vi "General Config.vi"(8 "error In":errorcluster, 10 "IOList":T2, 11 "reference":refnum<vi>) -> (0 "error out":errorcluster, 3 "Out reference":refnum<vi>)   [LabVIEW 2015]
uses:
  Control Button/Exit.ctl
  Control Button/Daq.ctl
  Control Button/Scanner config.ctl
  Control Button/Program Seq.ctl
  Control Button/cali.ctl
  Control Button/shift change.ctl
  Control Button/User mgt.ctl
  Control Button/model create.ctl
  Galobal variable_TI.vi
panel:
  in  "Setting":bool
  in  "image Setting":bool
  out "User Name 3":string
  in  "Model Create":T1
  in  "User Mgt":T3
  out "User Name 2":string
  in  "Shift":T4
  in  "Calibration":T5
  in  "IO List Update":bool
  out "error out 2":errorcluster
  in  "error in (no error)":errorcluster
  in  "Program Seq":T6
  in  "Scanner config":T7
  in  "DAQ Config":T8
  out "User Name":string
  in  "Exit":T9
  out "String":string
  out "appended path":path
  in  "Ring":u16(ring)
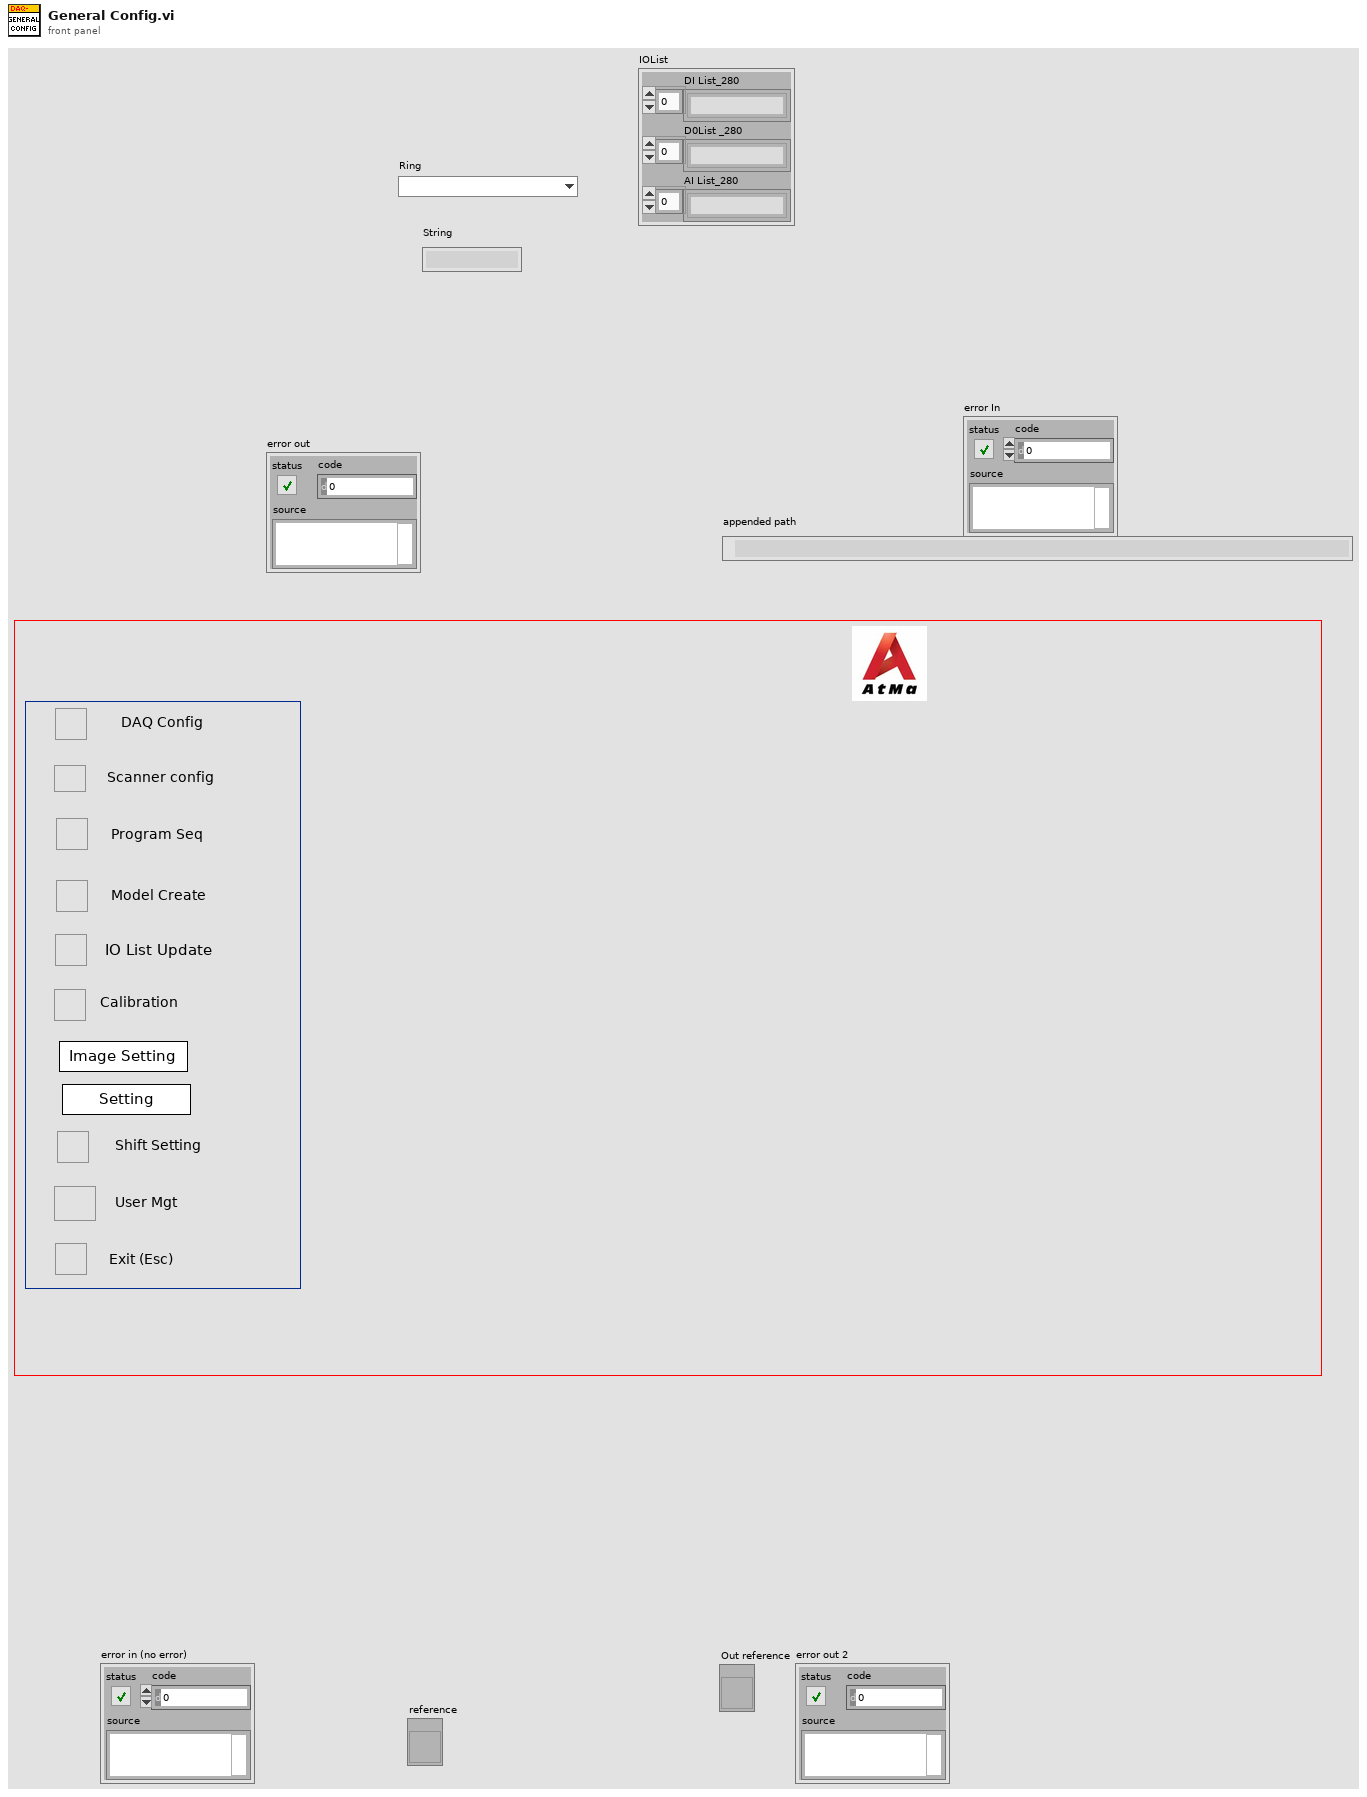
[diagram p1: front panel]
types:
  T1 = typedef "model create.ctl" = bool
  T2 = cluster{"DI List_280":string[], "D0List _280":string[], "AI List_280":string[]}
  T3 = typedef "User mgt.ctl" = bool
  T4 = typedef "shift change.ctl" = bool
  T5 = typedef "cali.ctl" = bool
  T6 = typedef "Program Seq.ctl" = bool
  T7 = typedef "Scanner config.ctl" = bool
  T8 = typedef "Daq.ctl" = bool
  T9 = typedef "Exit.ctl" = bool
  T10 = enum32{"Invalid", "Standard", "Closed", "Hidden", "Minimized", "Maximized"}
  T11 = cluster{"XInput":dbl[], "Y New Value":dbl[], "Avg point":i16}[]
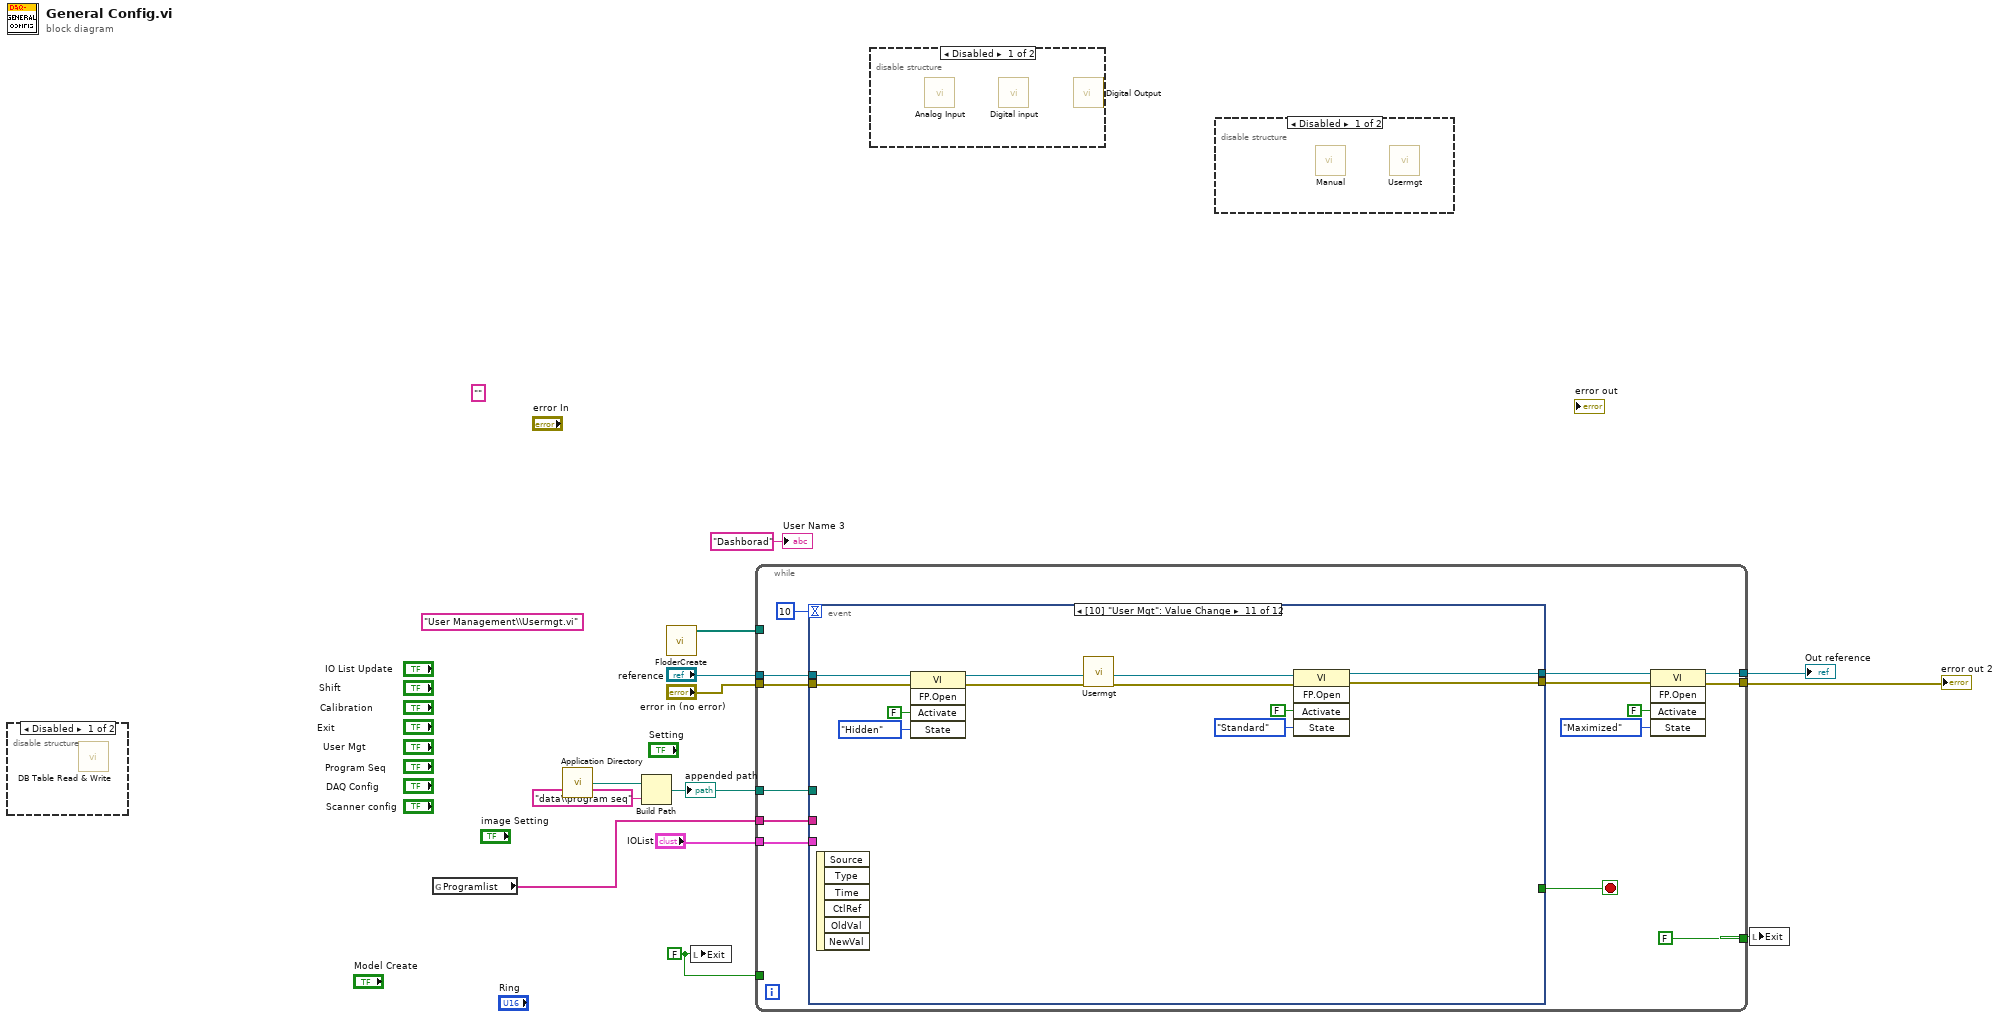
[diagram p0: block diagram]
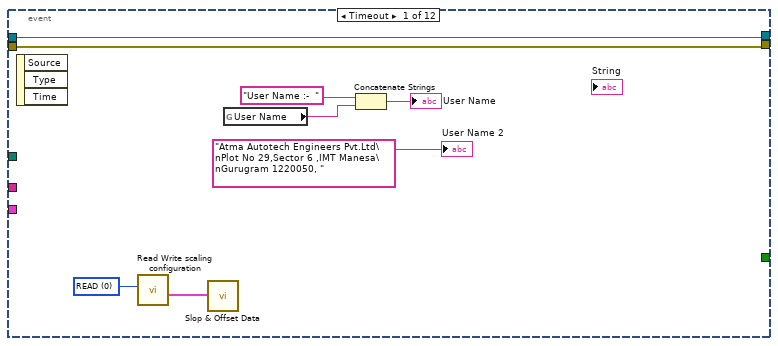
[diagram p5: hidden frame]
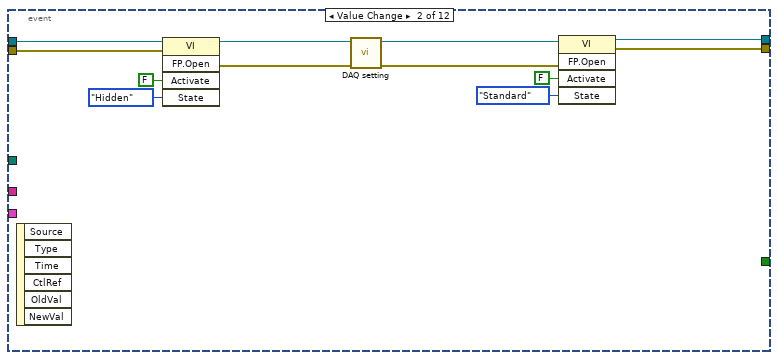
[diagram p6: hidden frame]
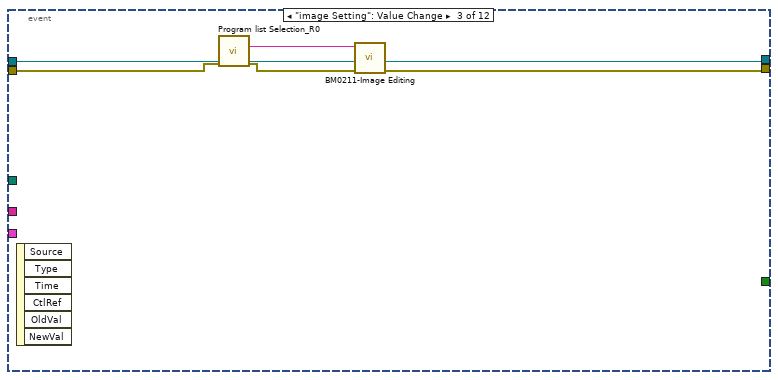
[diagram p7: hidden frame]
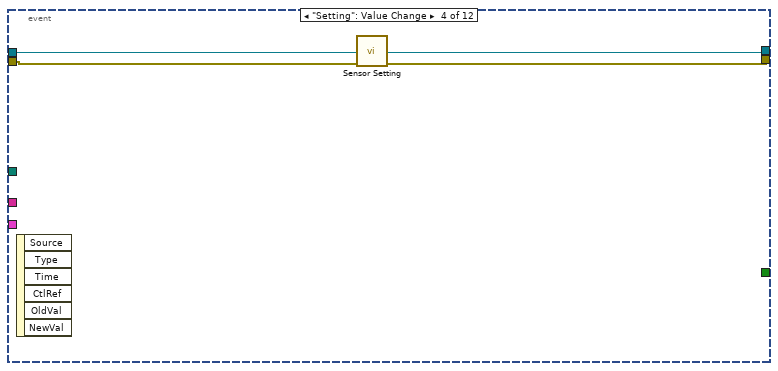
[diagram p8: hidden frame]
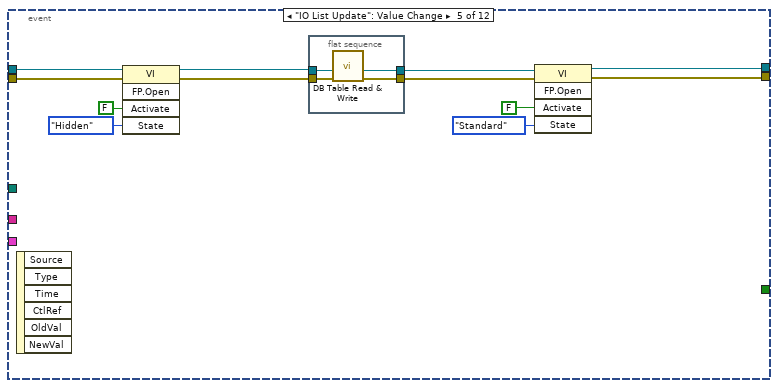
[diagram p9: hidden frame]
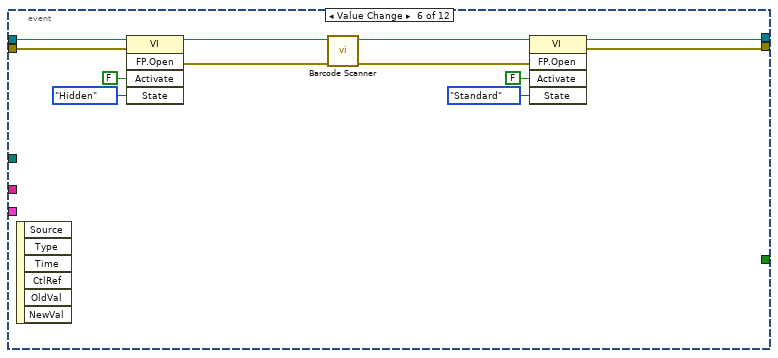
[diagram p10: hidden frame]
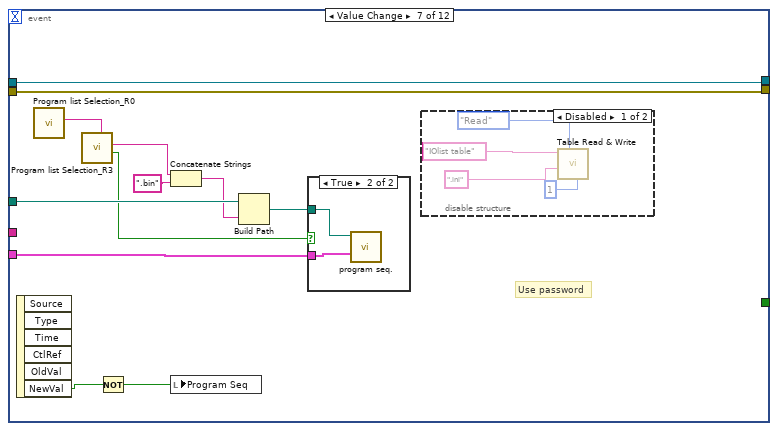
[diagram p11: hidden frame]
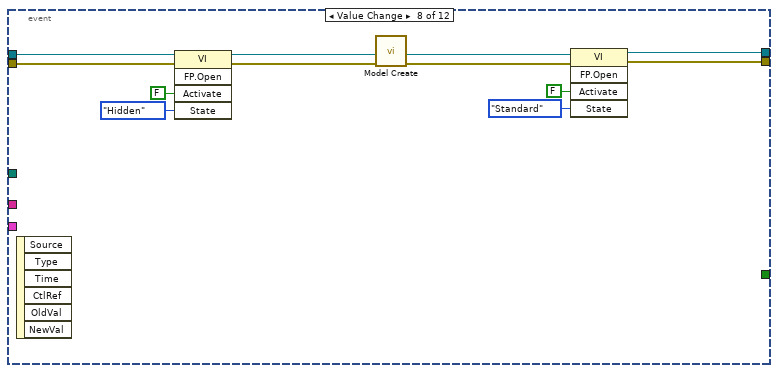
[diagram p14: hidden frame]
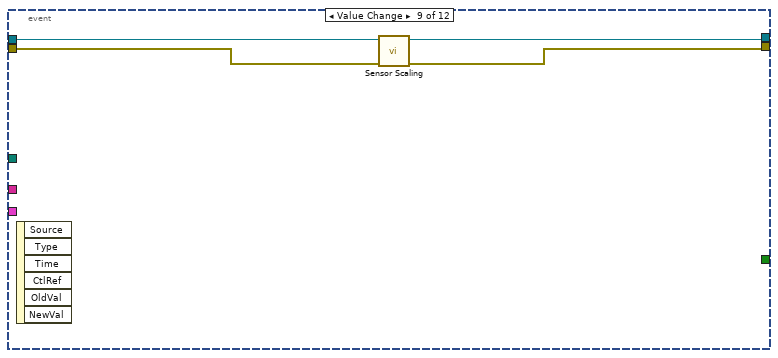
[diagram p15: hidden frame]
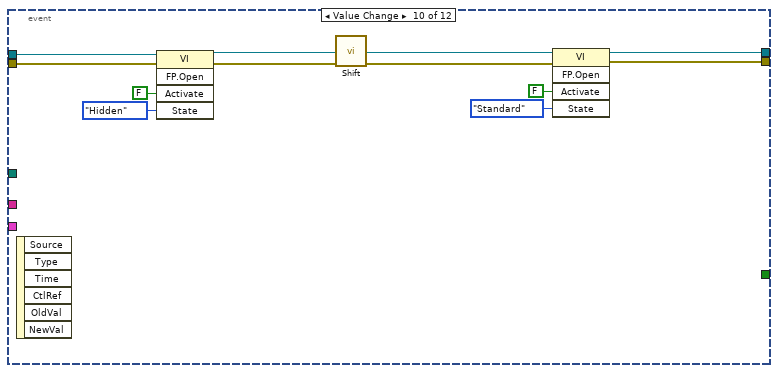
[diagram p16: hidden frame]
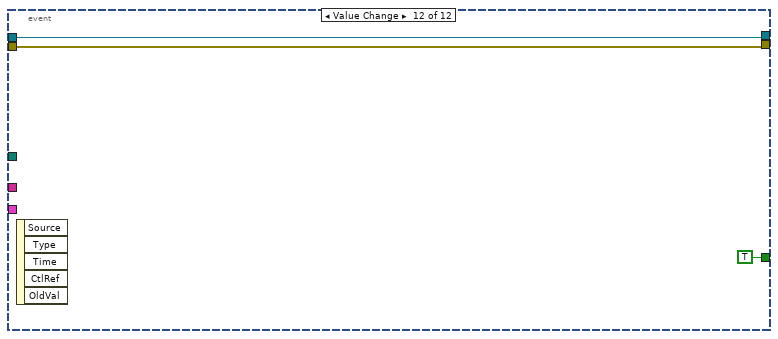
[diagram p17: hidden frame]
diagram:
  w10 = T9 FALSE ("Exit")
  (unwired) "User Management\\Usermgt.vi" ("name or relative path")
  (unwired) ""
  n1 = disable-structure shown="Disabled" {
    frame Disabled {
      n2 = call "DB Table Read & Write.vi"() -> ()  [unwired: 10 in, 2 out]
    }
    frame Enabled {
    }
  }
  n3 = global read "Galobal variable_TI.vi" "Programlist"() -> (w1:string[])
  n4 = call <vilib>:"Application Directory.vi"() -> ("Application Directory"=w6:path)
  n5 = Build Path(base path=w6, name or relative path="data\\program seq") -> (appended path=w3:path)
  "appended path" <- w3
  n6 = call "FloderCreate.vi"() -> ("File Path"=w7:path[])  [unwired: 11 in]
  n7 = local write "Exit"(w10) -> ()
  n8 = while {
    tunnel: w3 -> [w15]
    tunnel: "reference" -> [w25]
    tunnel: "error in (no error)" -> [w24]
    tunnel: [w19] -> w12
    tunnel: [w18] -> w11
    tunnel: w10 -> [_]
    tunnel: [T9 FALSE ("Exit")] -> w9
    tunnel: w7 -> [_]
    tunnel: "IOList" -> [w16]
    tunnel: w1 -> [w14]
    stop <- w26 stop-if-true
    n9 = event shown="[10] \"User Mgt\": Value Change" {
      selector: _ -> [_ _ _ _ _ _ _ _ _ _ _ _]
      dyn-events: _ -> [_ _ _ _ _ _ _ _ _ _ _ _]
      timeout: 10 -> [_ _ _ _ _ _ _ _ _ _ _ _]
      tunnel: [_ _ _ _ _ _ _ _ _ _ _ TRUE ("Exit")] -> w26
      tunnel: w25 -> [w32 w39 w52 w55 w59 w81 w95 w108 w115 w123 w132 w140]
      tunnel: w24 -> [w31 w38 w50 w54 w58 w80 w94 w107 w114 w121 w130 w139]
      tunnel: [w32 w37 w52 w55 w66 w73 w95 w103 w115 w122 w131 w140] -> w21
      tunnel: [w31 w36 w51 w53 w65 w72 w94 w102 w113 w120 w129 w139] -> w20
      tunnel: w16 -> [_ _ _ _ _ _ w93 _ _ _ _ _]
      tunnel: w15 -> [_ _ _ _ _ _ w92 _ _ _ _ _]
      tunnel: w14 -> [_ _ _ _ _ _ _ _ _ _ _ _]
      event Timeout {
        w30 = u16 0 items=["READ", "WRITE"] ("Read/Write")
        n10 = event-data() -> ()  [unwired: 1 in, 3 out]
        n11 = call "Read Write scaling configuration.vi"("Read/Write"=w30) -> ("Output"=w29:T11)  [unwired: 4 in, 2 out]
        n12 = call "Slop & Offset Data.vi"("Input"=w29) -> ()  [unwired: 10 in, 1 out]
        n13 = global read "Galobal variable_TI.vi" "User Name"() -> (w35:string)
        n14 = Concatenate Strings("User Name :-  " ("string"), w35) -> (→"User Name":string)
        "User Name 2" <- "Atma Autotech Engineers Pvt.Ltd\nPlot No 29,Sector 6 ,IMT Manesa\nGurugram 1220050, " ("string")
      }
      event Value Change {
        n15 = event-data() -> ()  [unwired: 1 in, 6 out]
        n16 = invoke class="VI" method="FP.Open"(reference=w39, error in=w38, "Activate"=FALSE ("Activate?"), "State"=T10."Hidden") -> (reference out=w45:refnum<vi>, error out=w44:errorcluster)  [unwired: 1 in, 3 out]
        n17 = call "DAQ setting.vi"("error in (no error)"=w44, "vi reference"=w45) -> ("error Out"=w40:errorcluster, "Out reference"=w41:refnum<vi>)  [unwired: 8 in]
        n18 = invoke class="VI" method="FP.Open"(reference=w41, error in=w40, "Activate"=FALSE ("Activate?"), "State"=T10."Standard") -> (reference out=w37:refnum<vi>, error out=w36:errorcluster)  [unwired: 1 in, 3 out]
      }
      event "image Setting": Value Change {
        n19 = event-data() -> ()  [unwired: 1 in, 6 out]
        n20 = call "Program list Selection_R0.vi"("error in"=w50) -> ("error out"=w49:errorcluster, "String"=w48:string)  [unwired: 7 in, 2 out]
        n21 = call "BM0211-Image Editing.vi"("error IN"=w49, "Running model"=w48) -> ("error out"=w51:errorcluster)  [unwired: 9 in]
      }
      event "Setting": Value Change {
        n22 = event-data() -> ()  [unwired: 1 in, 6 out]
        n23 = call "Sensor Setting.vi"("error in"=w54) -> ("error  out"=w53:errorcluster)  [unwired: 10 in]
      }
      event "IO List Update": Value Change {
        n24 = event-data() -> ()  [unwired: 1 in, 6 out]
        n25 = invoke class="VI" method="FP.Open"(reference=w59, error in=w58, "Activate"=FALSE ("Activate?"), "State"=T10."Hidden") -> (reference out=w57:refnum<vi>, error out=w56:errorcluster)  [unwired: 1 in, 3 out]
        n26 = flat-sequence {
          tunnel: [w68] -> w63
          tunnel: [w69] -> w62
          tunnel: w57 -> [w70]
          tunnel: w56 -> [w71]
          frame #0 {
            n27 = call "DB Table Read & Write.vi"("error in"=w71, "reference"=w70) -> ("error out"=w68:errorcluster, "referenceOut"=w69:refnum<vi>)  [unwired: 8 in]
          }
        }
        n28 = invoke class="VI" method="FP.Open"(reference=w62, error in=w63, "Activate"=FALSE ("Activate?"), "State"=T10."Standard") -> (reference out=w66:refnum<vi>, error out=w65:errorcluster)  [unwired: 1 in, 3 out]
      }
      event Value Change {
        n29 = event-data() -> ()  [unwired: 1 in, 6 out]
        n30 = invoke class="VI" method="FP.Open"(reference=w81, error in=w80, "Activate"=FALSE ("Activate?"), "State"=T10."Hidden") -> (reference out=w77:refnum<vi>, error out=w76:errorcluster)  [unwired: 1 in, 3 out]
        n31 = call "Barcode Scanner.vi"("error in (no error)"=w76, "reference"=w77) -> ("error in (no error) 2"=w74:errorcluster, "reference 2"=w75:refnum<vi>)  [unwired: 8 in]
        n32 = invoke class="VI" method="FP.Open"(reference=w75, error in=w74, "Activate"=FALSE ("Activate?"), "State"=T10."Standard") -> (reference out=w73:refnum<vi>, error out=w72:errorcluster)  [unwired: 1 in, 3 out]
      }
      event Value Change {
        # "Use password"
        n33 = event-data() -> ("NewVal"=w88:T6)  [unwired: 1 in, 5 out]
        n34 = call "Program list Selection_R0.vi"() -> ("String"=w86:string)  [unwired: 8 in, 3 out]
        n35 = call "Program list Selection_R3.vi"("new element/subarray"=w86) -> ("Exit"=w85:bool, "String"=w84:string)  [unwired: 7 in, 2 out]
        n36 = Not(x=w88) -> (.not. x?=w87:T6)
        n37 = Concatenate Strings(w84, ".bin" ("string")) -> (w91:string)
        n38 = local write "Program Seq"(w87) -> ()
        n39 = Build Path(base path=w92, name or relative path=w91) -> (appended path=w89:path)
        n40 = case shown="True" w85 {
          tunnel: w93 -> [_ w96]
          tunnel: w89 -> [_ w97]
          frame False {
          }
          frame True {
            n41 = call "program seq..vi"("IOList"=w96, "Filepath"=w97) -> ()  [unwired: 9 in, 1 out]
          }
        }
        n42 = disable-structure shown="Disabled" {
          frame Disabled {
            n43 = call "Table Read & Write.vi"("File Name"="IOlist table", "File type"=".ini", "Enum"=enum16{"Read", "Write"}."Read", "index"=1) -> ()  [unwired: 5 in, 2 out]
          }
          frame Enabled {
          }
        }
      }
      event Value Change {
        n44 = event-data() -> ()  [unwired: 1 in, 6 out]
        n45 = invoke class="VI" method="FP.Open"(reference=w108, error in=w107, "Activate"=FALSE ("Activate?"), "State"=T10."Hidden") -> (reference out=w104:refnum<vi>, error out=w106:errorcluster)  [unwired: 1 in, 3 out]
        n46 = call "Model Create.vi"("error in (no error)"=w106) -> ("error out"=w105:errorcluster)  [unwired: 10 in]
        n47 = invoke class="VI" method="FP.Open"(reference=w104, error in=w105, "Activate"=FALSE ("Activate?"), "State"=T10."Standard") -> (reference out=w103:refnum<vi>, error out=w102:errorcluster)  [unwired: 1 in, 3 out]
      }
      event Value Change {
        n48 = event-data() -> ()  [unwired: 1 in, 6 out]
        n49 = call "Sensor Scaling.vi"("error in"=w114) -> ("error out"=w113:errorcluster)  [unwired: 9 in, 1 out]
      }
      event Value Change {
        n50 = event-data() -> ()  [unwired: 1 in, 6 out]
        n51 = invoke class="VI" method="FP.Open"(reference=w123, error in=w121, "Activate"=FALSE ("Activate?"), "State"=T10."Hidden") -> (reference out=w124:refnum<vi>, error out=w126:errorcluster)  [unwired: 1 in, 3 out]
        n52 = call "Shift.vi"("error in"=w126) -> ("error out"=w125:errorcluster)  [unwired: 10 in]
        n53 = invoke class="VI" method="FP.Open"(reference=w124, error in=w125, "Activate"=FALSE ("Activate?"), "State"=T10."Standard") -> (reference out=w122:refnum<vi>, error out=w120:errorcluster)  [unwired: 1 in, 3 out]
      }
      event Value Change {
        n54 = event-data() -> ()  [unwired: 1 in, 6 out]
        n55 = invoke class="VI" method="FP.Open"(reference=w132, error in=w130, "Activate"=FALSE ("Activate?"), "State"=T10."Hidden") -> (reference out=w133:refnum<vi>, error out=w128:errorcluster)  [unwired: 1 in, 3 out]
        n56 = call "Usermgt.vi"("error In"=w128) -> ("error out"=w127:errorcluster)  [unwired: 10 in]
        n57 = invoke class="VI" method="FP.Open"(reference=w133, error in=w127, "Activate"=FALSE ("Activate?"), "State"=T10."Standard") -> (reference out=w131:refnum<vi>, error out=w129:errorcluster)  [unwired: 1 in, 3 out]
      }
      event Value Change {
        n58 = event-data() -> ()  [unwired: 1 in, 5 out]
      }
    }
    n59 = invoke class="VI" method="FP.Open"(reference=w21, error in=w20, "Activate"=FALSE ("Activate?"), "State"=T10."Maximized") -> (reference out=w19:refnum<vi>, error out=w18:errorcluster)  [unwired: 1 in, 3 out]
  }
  "Out reference" <- w12
  "error out 2" <- w11
  n60 = disable-structure shown="Disabled" {
    frame Disabled {
      n61 = call "Analog Input.vi"() -> ()  [unwired: 10 in, 2 out]
      n62 = call "Digital input.vi"() -> ()  [unwired: 10 in, 2 out]
      n63 = call "Digital Output.vi"() -> ()  [unwired: 10 in, 2 out]
    }
    frame Enabled {
    }
  }
  n64 = disable-structure shown="Disabled" {
    frame Disabled {
      n65 = call "Manual.vi"() -> ()  [unwired: 10 in, 2 out]
      n66 = call "Usermgt.vi"() -> ()  [unwired: 11 in, 1 out]
    }
    frame Enabled {
    }
  }
  n67 = local write "Exit"(w9) -> ()
  "User Name 3" <- "Dashborad" ("User Name 3")
